vi "Auto Shoot.vi"(4 "RPM Override?":i32, 6 "Angle Override?":i32, 8 "Angle":dbl, 9 "Right RPM":dbl, 10 "Left RPM":dbl, 11 "Shot Type":i32) -> (3 "Finished?":bool)   [LabVIEW 2015]
uses:
  Common Code/Catapult Auto Commands.ctl
  Common Code/Shoot Modes Enum.ctl
  Common Code/Shot Type.ctl
  Common Code/Drivetrain Modes.ctl
  Common Code/Change Detect Boolean.vi
  Robot Global Data.vi
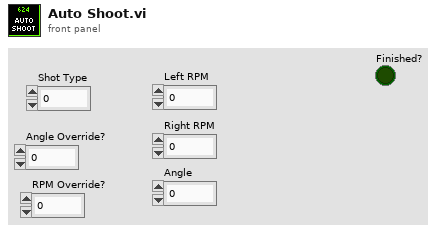
[diagram p1: front panel]
types:
  T1 = typedef "Catapult Auto Commands.ctl" = enum16{"Idle", "Warmup", "Shoot"}
  T2 = typedef "Drivetrain Commands.ctl" = cluster{"Y Power":dbl, "Turn Power":dbl, "2nd Gear?":bool, "Modes":T3, "Heading Target":dbl, "X Max Speed":dbl, "Y Max Speed":dbl, "X Min Speed":dbl, "Y Min Speed":dbl, "Y Target":dbl, "Max Accel":dbl, "Max Velocity":dbl, "Y Power 2":dbl, "Pivot Speed":dbl}
  T3 = typedef "Drivetrain Modes.ctl" = enum16{"Tank", "Climb", "Manual", "Goal Vision Targeting", "PID Distance Drive", "Hybrid", "Gyro Steer"}
  T4 = typedef "Shoot Modes Enum.ctl" = enum16{"Manual", "Auto"}
  T5 = typedef "Shot Type.ctl" = enum16{"Batter Shot", "Corner Shot", "Cleat Shot", "Vision Shot", "Deep Middle Shot"}
  T6 = typedef "Manual Shoot.ctl" = cluster{"Spin Wheels":bool, "Fire":bool, "Angle":dbl, "Angle Power":dbl, "Use Manual Angle":bool, "Override RPM":bool, "Left RPM":dbl, "Right RPM":dbl, "Secure Ball?":bool}
  T7 = typedef "Shooter State Cluster.ctl" = cluster{"State":T8, "Left RPM":dbl, "Right RPM":dbl, "Shooter Ready?":bool, "Ball Loaded?":bool, "Current Angle":dbl, "Angle Motor Output":dbl, "Trigger Output":dbl, "Angle Ready?":bool, "RPM Ready?":bool, "Vision Ready?":bool, "Ball Loaded?":bool, "Mode":T4, "Shot Type":T5, "Pot Height":dbl, "Current Tripped Forward?":bool, "Current Tripped Backward?":bool, "Right Servo":i32, "Left Servo":i32, "IR Override":bool, "Intake Danger?":bool, "Intake Angle Ready?":bool}
  T8 = typedef "Shooter State.ctl" = enum16{"Idle", "Settle Ball", "Warmup", "Shooter Ready", "Shoot"}
  T9 = typedef "Shooter Command Cluster.ctl" = cluster{"Command":T1, "Mode":T4, "Shot Type":T5, "Override Trigger Sensor":bool, "Override Angle?":bool, "Hide From Death":bool}
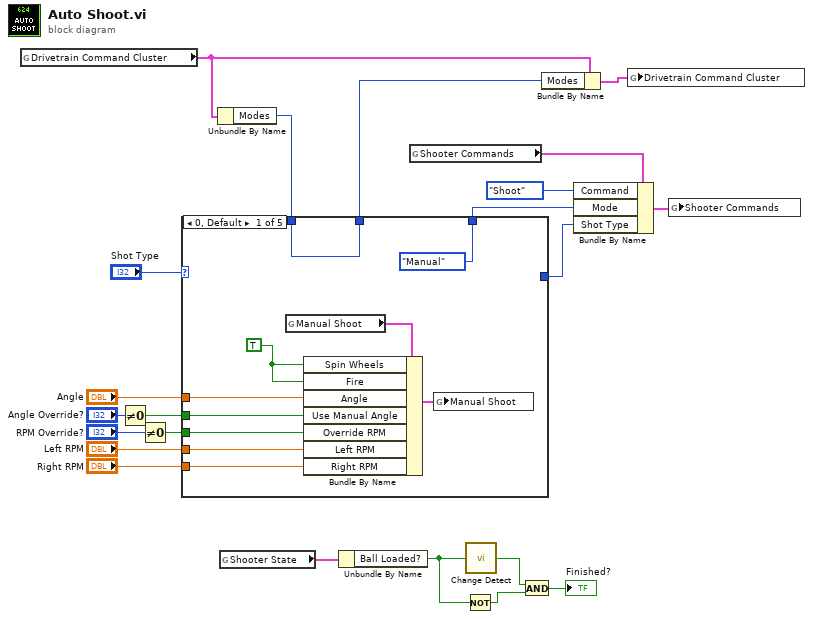
[diagram p0: block diagram]
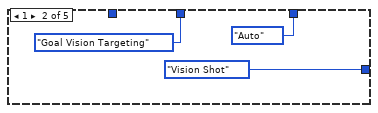
[diagram p2: hidden frame]
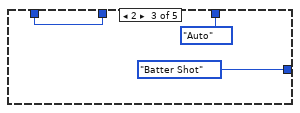
[diagram p3: hidden frame]
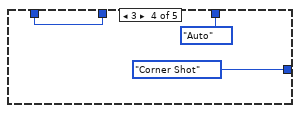
[diagram p4: hidden frame]
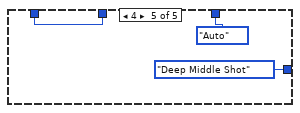
[diagram p5: hidden frame]
diagram:
  n1 = global read "Robot Global Data.vi" "Drivetrain Command Cluster"() -> (w2:T2)
  n2 = Not Equal To 0?(x="Angle Override?") -> (x != 0?=w13:bool)
  n3 = Not Equal To 0?(x="RPM Override?") -> (x != 0?=w15:bool)
  n4 = Unbundle By Name(w2) -> ("Modes"=w1:T3)
  n5 = case shown="0, Default" "Shot Type" {
    tunnel: [Shoot_Modes_Enum."Manual" ("Mode") Shoot_Modes_Enum."Auto" ("Mode") Shoot_Modes_Enum."Auto" ("Mode") Shoot_Modes_Enum."Auto" ("Mode") Shoot_Modes_Enum."Auto" ("Mode")] -> w19
    tunnel: [_ Shot_Type."Vision Shot" ("Shot Type") Shot_Type."Batter Shot" ("Shot Type") Shot_Type."Corner Shot" ("Shot Type") Shot_Type."Deep Middle Shot" ("Shot Type")] -> w18
    tunnel: w15 -> [w28 _ _ _ _]
    tunnel: w13 -> [w27 _ _ _ _]
    tunnel: "Left RPM" -> [w26 _ _ _ _]
    tunnel: "Right RPM" -> [w25 _ _ _ _]
    tunnel: "Angle" -> [w24 _ _ _ _]
    tunnel: [w23 Drivetrain_Modes."Goal Vision Targeting" ("Modes") w36 w39 w42] -> w3
    tunnel: w1 -> [w23 _ w36 w39 w42]
    frame 0, Default {
      w30 = TRUE ("Spin Wheels")
      n6 = global read "Robot Global Data.vi" "Manual Shoot"() -> (w32:T6)
      n7 = Bundle By Name(cluster=w32, "Spin Wheels"=w30, "Fire"=w30, "Angle"=w24, "Use Manual Angle"=w27, "Override RPM"=w28, "Left RPM"=w26, "Right RPM"=w25) -> (w29:T6)
      n8 = global write "Robot Global Data.vi" "Manual Shoot"(w29) -> ()
    }
    frame 1 {
    }
    frame 2 {
    }
    frame 3 {
    }
    frame 4 {
    }
  }
  n9 = global read "Robot Global Data.vi" "Shooter State"() -> (w9:T7)
  n10 = Unbundle By Name(w9) -> ("Ball Loaded?"=w8:bool)
  n11 = global read "Robot Global Data.vi" "Shooter Commands"() -> (w22:T9)
  n12 = Not(x=w8) -> (.not. x?=w7:bool)
  n13 = call-poly "Change Detect.vi"("In"=w8) -> ("Changed?"=w6:bool)
  n14 = And(x=w6, y=w7) -> (x .and. y?=→"Finished?":bool)
  n15 = Bundle By Name(cluster=w2, "Modes"=w3) -> (w4:T2)
  n16 = Bundle By Name(cluster=w22, "Command"=Catapult_Auto_Commands."Shoot", "Mode"=w19, "Shot Type"=w18) -> (w17:T9)
  n17 = global write "Robot Global Data.vi" "Drivetrain Command Cluster"(w4) -> ()
  n18 = global write "Robot Global Data.vi" "Shooter Commands"(w17) -> ()
